vi "input.vi"(8 "error in":errorcluster, 10 "data table in":T1, 11 "J1939 runtime in":refnum<class "J1939 runtime.lvclass">) -> (0 "error out":errorcluster, 2 "data table out":T1, 3 "J1939 runtime out":refnum<class "J1939 runtime.lvclass">)   [LabVIEW 2014, in "J1939 runtime.lvclass"]
doc: "Provides an interface for reading data from a module at runtime. While this interface performs no operations, a child should provide an override which may read from any open sessions, references, or interfaces."
uses:
  J1939 runtime.lvclass
  <vilib>/NI/Tag Bus/table/data table.ctl
  J1939 runtime.lvclass/J1939 runtime.ctl
  <vilib>/xnet/xnet.llb/XNET Read (Signal Single-point).vi
  <vilib>/NI/Tag Bus/table/data table.lvlib
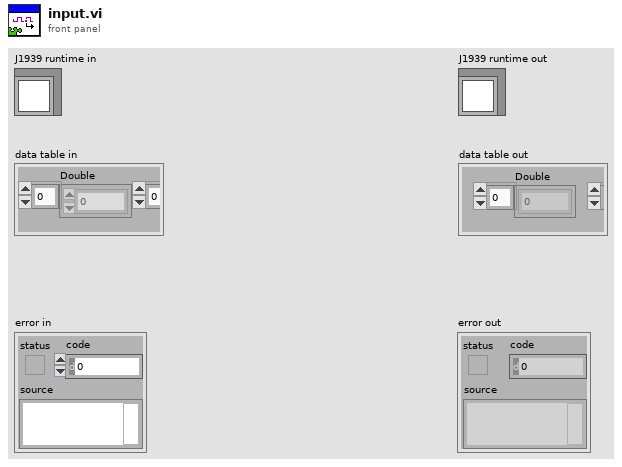
[diagram p1: front panel]
types:
  T1 = typedef "tag bus.lvlib/data table.lvlib/data table.ctl" = cluster{"Double":dbl[], "Single":sgl[], "I64":i64[], "I32":i32[], "I16":i16[], "I8":i8[], "U64":u64[], "U32":u32[], "U16":u16[], "U8":u8[], "Boolean":bool[], "String":string[], "Array of Double":cluster{"DBL Array":dbl[]}[], "Array of Single":cluster{"SGL Array":sgl[]}[], "Array of I64":cluster{"I64 Array":i64[]}[], "Array of I32":cluster{"I32 Array":i32[]}[], "Array of I16":cluster{"I16 Array":i16[]}[], "Array of I8":cluster{"I8 Array":i8[]}[], "Array of U64":cluster{"U64 Array":u64[]}[], "Array of U32":cluster{"U32 Array":u32[]}[], "Array of U16":cluster{"U16 Array":u16[]}[], "Array of U8":cluster{"U8 Array":u8[]}[], "Array of Boolean":cluster{"Boolean Array":bool[]}[], "Array of String":cluster{"String Array":string[]}[]}
  T2 = typedef "J1939 configuration.lvclass/Signal Mapping.ctl" = cluster{"data type":T3, "index":i32}
  T3 = typedef "tag bus.lvlib/tag descriptor.lvclass/Data Type.ctl" = enum16{"Double", "Single", "I64", "I32", "I16", "I8", "U64", "U32", "U16", "U8", "Boolean", "String", "Array of Double", "Array of Single", "Array of I64", "Array of I32", "Array of I16", "Array of I8", "Array of U64", "Array of U32", "Array of U16", "Array of U8", "Array of Boolean", "Array of String"}
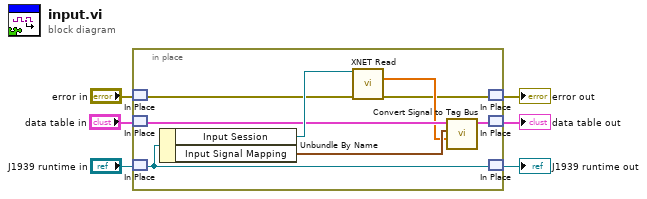
[diagram p0: block diagram]
diagram:
  n1 = in-place {
    n2 = in-place-match #1("error in") -> (w8:errorcluster)
    n3 = in-place-match #2("data table in") -> (w12:T1)
    n4 = in-place-match #3("J1939 runtime in") -> (w14:refnum<class "J1939 runtime.lvclass">)
    n5 = Unbundle By Name(w14) -> ("Input Session"=w13:refnum<k21>, "Input Signal Mapping"=w10:T2[])
    n6 = call-poly <vilib>:"XNET Read.vi"("session in"=w13, "error in (no error)"=w8) -> ("data"=w9:dbl[], "error out"=w7:errorcluster)  [unwired: 12 out]
    n7 = call "Convert Signal to Tag Bus.vi"("Signals"=w9, "signal mapping"=w10, "data table in in"=w12) -> ("data table out 2"=w11:T1)  [unwired: 8 in]
    n8 = in-place-match #1(w7) -> (→"error out":errorcluster)
    n9 = in-place-match #2(w11) -> (→"data table out":T1)
    n10 = in-place-match #3(w14) -> (→"J1939 runtime out":refnum<class "J1939 runtime.lvclass">)
  }
